vi "Configure.vi"(8 "error in (no error)":errorcluster, 11 "navX - SPI in":refnum<class "navX - SPI.lvclass">) -> (0 "error out":errorcluster, 3 "navX - SPI out":refnum<class "navX - SPI.lvclass">)   [LabVIEW 2015, in "navX Library v3.lvlib" / "navX - SPI.lvclass"]
uses:
  navX - SPI.lvclass
  navX - Base/navX - Base.lvclass
  navX - Base/DeviceRegistryTypeDef.ctl
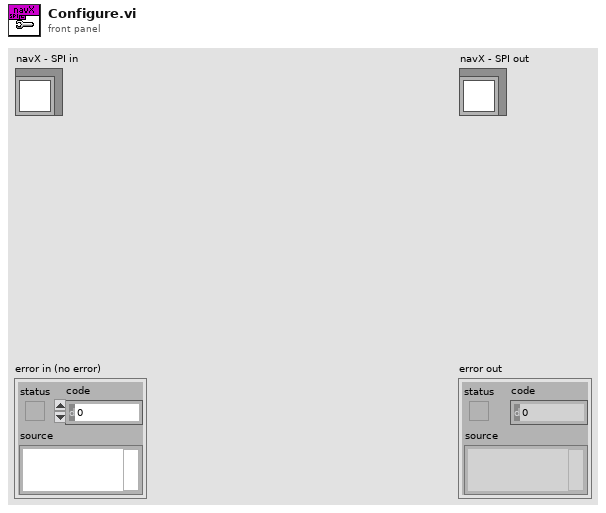
[diagram p1: front panel]
types:
  T1 = typedef "navX Library v3.lvlib/navX - Base.lvclass/DeviceRegistryTypeDef.ctl" = u8
  T2 = typedef "WPI_SPIDevRef.ctl" = cluster{"DevStatus":errorcluster, "Handle":i32, "SPI Bus":T3}
  T3 = typedef "spi_bus.ctl" = enum16{"SPI On-Board, CS0", "SPI On-Board, CS1", "SPI On-Board, CS2", "SPI On-Board, CS3", "SPI MXP", "Invalid"}
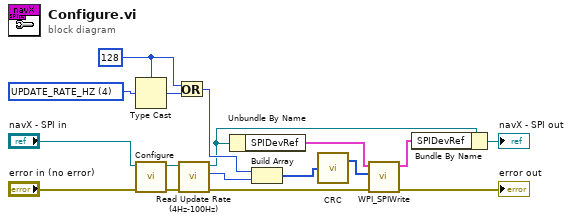
[diagram p0: block diagram]
diagram:
  w12 = u8 128
  w11 = T1 4 items=["WHOAMI"=0, "HW_REV"=1, "FW_VER_MAJOR"=2, "FW_VER_MINOR"=3, "UPDATE_RATE_HZ"=4, "ACCEL_FSR_G"=5, "GYRO_FSR_DPS"=6, "OP_STATUS"=8, "CAL_STATUS"=9, "SELFTEST_STATUS"=10, "CAPABILITY_FLAGS_L"=11, "CAPABILITY_FLAGS_H"=12, "SENSOR_STATUS"=16, "TIMESTAMP"=18, "YAW"=22, "ROLL"=24, "PITCH"=26, "HEADING"=28, "FUSED_HEADING"=30, "ALTITUDE_I"=32, "ALTITUDE_D"=34, "LINERA_ACC_X"=36, "LINERA_ACC_Y"=38, "LINERA_ACC_Z"=40, "QUAT_W"=42, "QUAT_X"=44, "QUAT_Y"=46, "QUAT_Z"=48, "MPU_TEMP_C"=50, "GYRO_X"=52, "GYRO_Y"=54, "GYRO_Z"=56, "ACC_X"=58, "ACC_Y"=60, "ACC_Z"=62, "MAG_X"=64, "MAG_Y"=66, "MAG_Z"=68, "PRESSURE_I"=70, "PRESSURE_D"=72, "PRESSURE_TEMP"=74, "YAW_OFFSET"=76, "QUAT_OFFSET_W"=78, "QUAT_OFFSET_X"=80, "QUAT_OFFSET_Y"=82, "QUAT_OFFSET_Z"=84, "INTEGRATION_CONTROL"=86, "VELOCITY_X"=88, "VELOCITY_Y"=92, "VELOCITY_Z"=96, "DISPLACMENT_X"=100, "DISPLACMENT_Y"=104, "DISPLACEMENT_Z"=108] ("Device Register")
  n1 = Type Cast(type=w12, x=w11) -> (*(type *) &x=w13:u8)
  n2 = call-parent "Configure.vi"("error in (no error)"="error in (no error)", "navX - Base in"="navX - SPI in") -> ("error out"=w14:errorcluster, "navX - Base out"=w15:refnum<class "navX - SPI.lvclass">)  [unwired: 8 in]
  n3 = Or(x=w12, y=w13) -> (x .or. y?=w10:u8)
  n4 = call "Read Update Rate (4Hz-100Hz).vi"("error in (no error)"=w14, "navX - Base in"=w15) -> ("error out"=w1:errorcluster, "Update Rate (4Hz-100Hz)"=w9:u8, "navX - Base out"=w6:refnum<class "navX - SPI.lvclass">)  [unwired: 6 in, 1 out]
  n5 = Unbundle By Name(w6) -> ("SPIDevRef"=w4:T2)
  n6 = Build Array(w10, w9) -> (w8:u8[])
  n7 = call "CRC.vi"("Message"=w8) -> ("Message with CRC"=w7:u8[])  [unwired: 1 out]
  n8 = call <vilib>:"WPI_SPIWrite.vi"("error in (no error)"=w1, "Data To Send"=w7, "SPIDevRef"=w4) -> ("error out"=→"error out":errorcluster, "SPIDevRef"=w3:T2)  [unwired: 6 in, 1 out]
  n9 = Bundle By Name(cluster=w6, "SPIDevRef"=w3) -> (→"navX - SPI out":refnum<class "navX - SPI.lvclass">)
